vi "Get Number Pre Amp Gains.vi"(11 "noGains":i32) -> (2 "function return":u32, 3 "noGains out":i32)   [LabVIEW 2018, in "AndorSDK.lvlib"]
doc: "EXPNETTYPE unsigned int WINAPI GetNumberPreAmpGains(int * noGains);"
uses:
  AndorSDK.lvlib
  ATMCD32D.dll
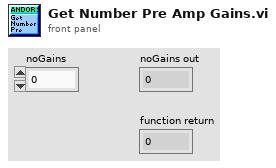
[diagram p1: front panel]
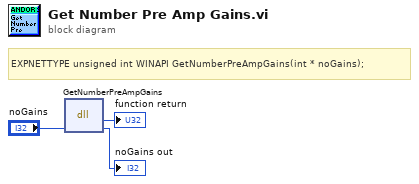
[diagram p0: block diagram]
diagram:
  # "EXPNETTYPE unsigned int WINAPI GetNumberPreAmpGains(int * noGains);"
  n1 = dll-call lib="PTH2babs E\nPersönliches02 - Arbeit03-HiwijobsLabviewCodelibANDOR\tAndor SDK\nATMCD32D.*" fn="GetNumberPreAmpGains"("noGains"="noGains") -> (→"function return":u32, "noGains"=→"noGains out":i32)  [unwired: 3 in, 2 out]
